vi "read.vi"(8 "error in (no error)":errorcluster, 11 "SerialConnection in":refnum<class "SerialConnection.lvclass">) -> (0 "error out":errorcluster, 2 "message":string, 3 "SerialConnection out":refnum<class "SerialConnection.lvclass">)   [LabVIEW 2023, in "AbstractFactory.lvlib" / "SerialConnection.lvclass"]
uses:
  SerialConnection.lvclass
  SerialConnection.lvclass/SerialConnection.ctl
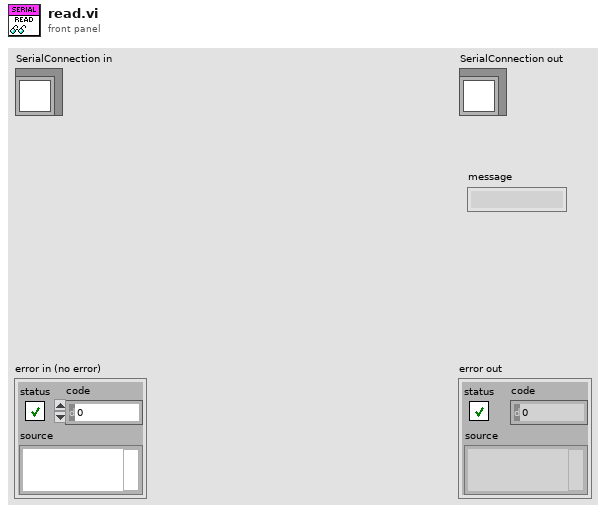
[diagram p1: front panel]
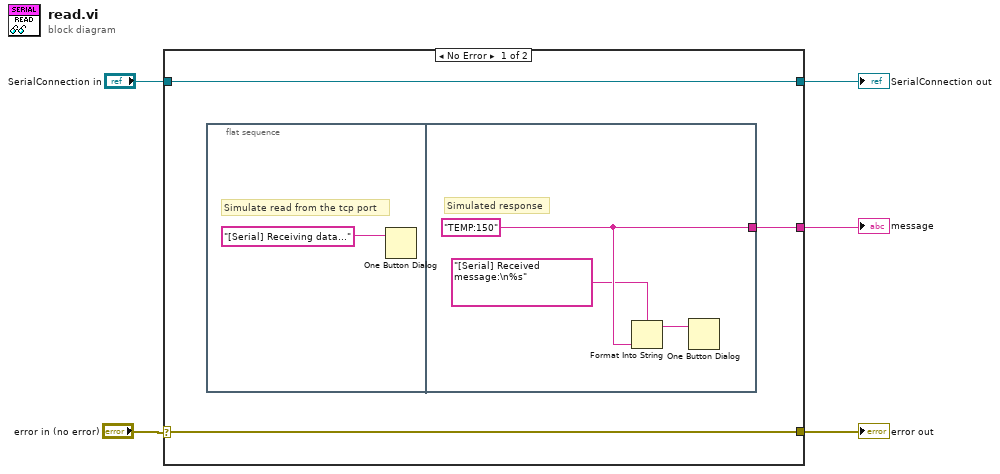
[diagram p0: block diagram]
diagram:
  n1 = case shown="No Error" "error in (no error)" {
    selector: "error in (no error)" -> [w7 w13]
    tunnel: "SerialConnection in" -> [w8 w14]
    tunnel: [w8 w14] -> w3
    tunnel: [w7 w13] -> w2
    tunnel: [w6 _] -> w1
    frame No Error {
      n2 = flat-sequence {
        tunnel: [w12] -> w6
        frame #0 {
          # "Simulate read from the tcp port"
          n3 = One Button Dialog(message="[Serial] Receiving data..." ("format string")) -> ()  [unwired: 1 in, 1 out]
        }
        frame #1 {
          w12 = "TEMP:150" ("message")
          # "Simulated response"
          n4 = Format Into String(format string="[Serial] Received message:\n%s", w12) -> (resulting string=w10:string)  [unwired: 2 in, 1 out]
          n5 = One Button Dialog(message=w10) -> ()  [unwired: 1 in, 1 out]
        }
      }
    }
    frame Error {
    }
  }
  "error out" <- w2
  "SerialConnection out" <- w3
  "message" <- w1
